vi "_Add App.vi"(8 "error in (no error)":errorcluster, 11 "App in":refnum<class "App.lvclass">) -> (0 "error out":errorcluster, 3 "App out":refnum<class "App.lvclass">)   [LabVIEW 2020, in "PicoG-App.lvlib" / "App.lvclass"]
uses:
  App.lvclass
  ViaApp/ViaApp.lvclass
  App Watcher/App Watcher.lvclass
  AppListPanel/AppListPanel.lvclass
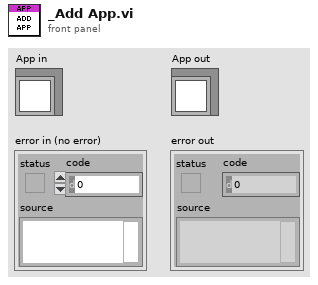
[diagram p1: front panel]
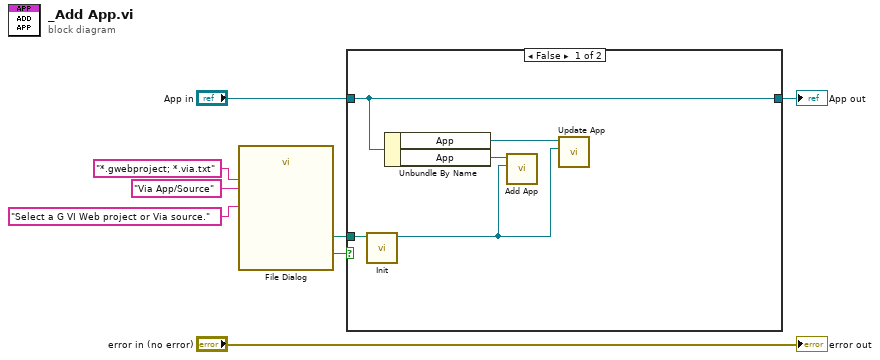
[diagram p0: block diagram]
diagram:
  n1 = call "File Dialog"("prompt"="Select a G VI Web project or Via source.", "pattern (all files)"="*.gwebproject; *.via.txt", "pattern label"="Via App/Source") -> ("selected path"=w2:path, "cancelled"=w3:bool)  [unwired: 9 in, 2 out]
  n2 = case shown="False" w3 {
    tunnel: "App in" -> [w9 w14]
    tunnel: w2 -> [w13 _]
    tunnel: [w9 w14] -> w1
    frame False {
      n3 = call "Init.vi"("Path"=w13) -> ("ViaApp out"=w10:refnum<class "ViaApp.lvclass">)  [unwired: 9 in, 1 out]
      n4 = Unbundle By Name(w9) -> ("App"=w11:refnum<class "AppListPanel.lvclass">, "App"=w12:refnum<class "App Watcher.lvclass">)
      n5 = call "Add App.vi"("ViaApp"=w10, "App Watcher in"=w12) -> ()  [unwired: 8 in, 2 out]
      n6 = call "Update App.vi"("ViaApp"=w10, "AppListPanel in"=w11) -> ()  [unwired: 8 in, 2 out]
    }
    frame True {
    }
  }
  "App out" <- w1
  "error out" <- "error in (no error)"
